vi "Modify Button.vi"(8 "error in (no error)":errorcluster, 10 "Array":path[](array[path]), 11 "ctl in":refnum<class "ctl.lvclass">) -> (0 "error out":errorcluster, 3 "ctl out":refnum<class "ctl.lvclass">)   [LabVIEW 2012, in "ctl.lvclass"]
uses:
  ctl.lvclass
  ctl.lvclass/ctl.ctl
  _ResManager_v86/IDCloneResMgr.lvlib
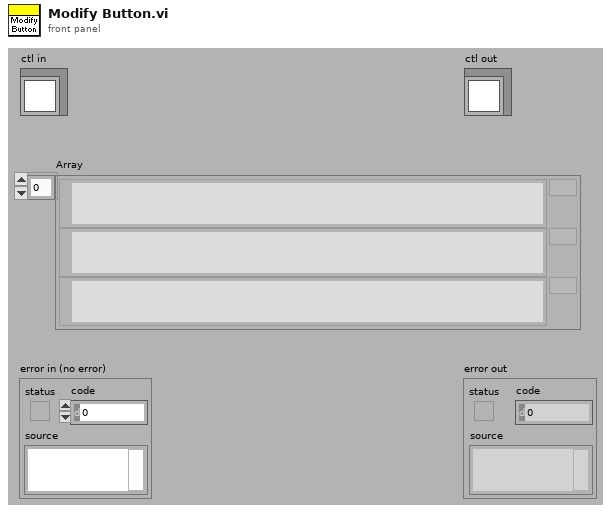
[diagram p1: front panel]
types:
  T1 = cluster{"type":u32, "id":i32, "name":string, "binary data":string}[]
  T2 = typedef "IDCloneResMgr.lvlib/IDClone_Resource info.ctl" = cluster{"type":u32, "id":i32, "name":string, "binary data":string}
  T3 = typedef "IDCloneResMgr.lvlib/ID_Resource info.ctl" = cluster{"type":u32, "id":i32, "name":string, "binary data":string}
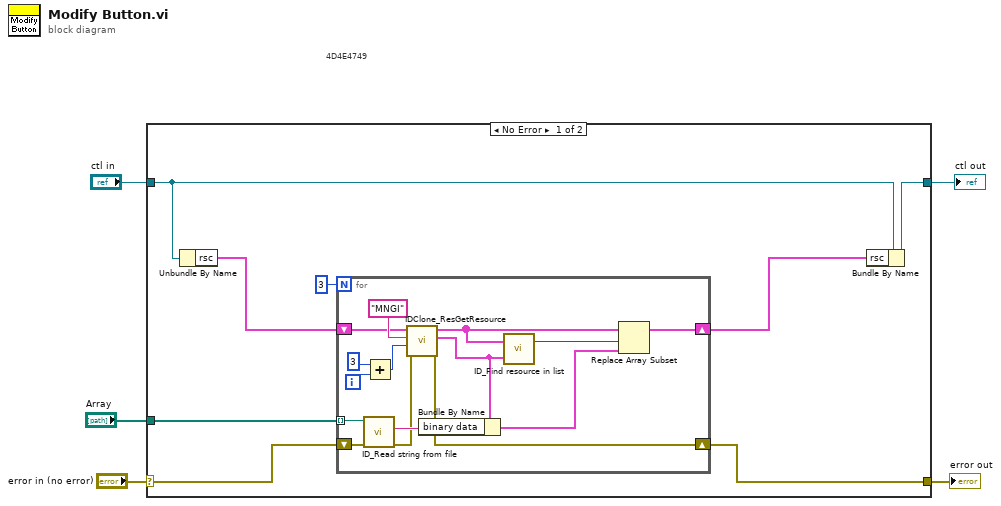
[diagram p0: block diagram]
diagram:
  # "4D4E4749"
  n1 = case shown="No Error" "error in (no error)" {
    selector: "error in (no error)" -> [w7 w30]
    tunnel: [w6 w30] -> w3
    tunnel: [w12 w29] -> w2
    tunnel: "ctl in" -> [w13 w29]
    tunnel: "Array" -> [w9 _]
    frame No Error {
      n2 = Unbundle By Name(w13) -> ("rsc"=w10:T1)
      n3 = for {
        N: 3 -> [_]
        shift-right: [w24] -> w11
        shift-left: w10 -> [w25]
        tunnel: w9 -> [w19] mode=indexing
        shift-right: [w14] -> w6
        shift-left: w7 -> [w16]
        i -> [w23]
        n4 = call "ID_Read string from file.vi"("error in (no error)"=w16, "path"=w19) -> ("error out"=w15:errorcluster, "string"=w18:string)  [unwired: 3 in, 5 out]
        n5 = Add(x=3 ("id"), y=w23) -> (x+y=w17:i32)
        n6 = call "IDClone_ResGetResource.vi"("error in (no error)"=w15, "id"=w17, "type"="MNGI" ("type string"), "resources"=w25) -> ("error out"=w14:errorcluster, "resource info"=w21:T2, "resources"=w27:T3[])  [unwired: 5 out]
        n7 = Bundle By Name(cluster=w21, "binary data"=w18) -> (w20:T2)
        n8 = call "ID_Find resource in list.vi"("info to match"=w21, "resources"=w27) -> ("index"=w28:i32)  [unwired: 1 out]
        n9 = Replace Array Subset(array=w27, new element=w20, index=w28) -> (w24:T3[])
      }
      n10 = Bundle By Name(cluster=w13, "rsc"=w11) -> (w12:refnum<class "ctl.lvclass">)
    }
    frame Error {
    }
  }
  "error out" <- w3
  "ctl out" <- w2
